vi "Stop Core.vi"(10 "final error code":i32, 11 "Stepper in":refnum<class "Stepper.lvclass">) -> (3 "Stepper out":refnum<class "Stepper.lvclass">)   [LabVIEW 2015, in "Stepper.lvclass"]
doc: "(<B>Filename</B>: Actor Framework.lvlib:Actor.lvclass:Stop Core.vi)\n\nDefines what the actor does before it stops. Use the <B>final error code</B> input to determine whether the actor shut down in response to an error.\n\nBy default, this method does nothing. A descendant class may override it to define behavior, such as shutting down any processes the actor initiated in its override of the Actor Core method."
uses:
  Stepper.lvclass
  Stepper.lvclass/Stepper.ctl
  CO2 Actor/CO2 Actor.lvclass
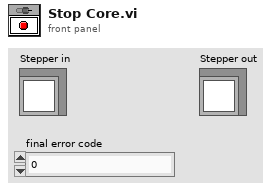
[diagram p1: front panel]
types:
  T1 = cluster{"Syringe Vacuum Gauge":refnum<k21>, "Setpoint":refnum<k21>, "SM Ticks":refnum<k21>, "Enabled":refnum<k21>, "Home":refnum<k21>, "Run":refnum<k21>}
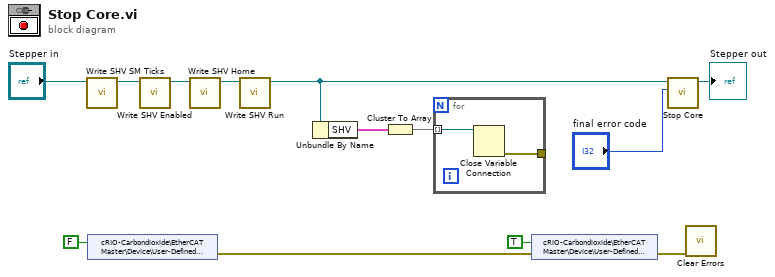
[diagram p0: block diagram]
diagram:
  n1 = call "Write SHV SM Ticks.vi"("Stepper in"="Stepper in") -> ("Stepper out"=w5:refnum<class "Stepper.lvclass">)  [unwired: 9 in, 1 out]
  n2 = shared-variable "cRIO-Carbondioxide\\EtherCAT Master\\Device\\User-Defined Variables\\SM Enable Drive"(FALSE ("Enable Drive")) -> (error out=w11:errorcluster)  [unwired: 1 in]
  n3 = call "Write SHV Enabled.vi"("Stepper in"=w5) -> ("Stepper out"=w3:refnum<class "Stepper.lvclass">)  [unwired: 9 in, 1 out]
  n4 = call "Write SHV Home.vi"("Stepper in"=w3) -> ("Stepper out"=w2:refnum<class "Stepper.lvclass">)  [unwired: 9 in, 1 out]
  n5 = call "Write SHV Run.vi"("Stepper in"=w2) -> ("Stepper out"=w1:refnum<class "Stepper.lvclass">)  [unwired: 9 in, 1 out]
  n6 = Unbundle By Name(w1) -> ("SHV"=w7:T1)
  n7 = Cluster To Array(cluster=w7) -> (array=w6:refnum<k21>[])
  n8 = for {
    tunnel: w6 -> [w15] mode=indexing
    tunnel: [w14] -> _
    n9 = Close Variable Connection(11:w15) -> (0:w14:errorcluster)  [unwired: 1 in]
  }
  n10 = shared-variable "cRIO-Carbondioxide\\EtherCAT Master\\Device\\User-Defined Variables\\SM Clear Faults"(TRUE ("Clear Faults"), error in=w11) -> (error out=w4:errorcluster)
  n11 = call-parent "Stop Core.vi"("final error code"="final error code", "CO2 Actor in"=w1) -> ("CO2 Actor out"=→"Stepper out":refnum<class "Stepper.lvclass">)  [unwired: 9 in]
  n12 = call <vilib>:"Clear Errors.vi"("error in (no error)"=w4) -> ()  [unwired: 5 in, 2 out]
